vi "UnregisterMat_1DArray-CXT.vi"(6 "AdressOrData":cxt[](array[numeric]), 8 "error in":errorcluster, 11 "Image":u8) -> (0 "error out":errorcluster, 3 "Datatype":cxt[](array[numeric]))   [LabVIEW 2020, in "OpenLvVision_OpenCv.lvlib"]
doc: "Register mat for dll.\nNo malleable to breake vi inlining!"
uses:
  OpenLvVision_OpenCv.lvlib
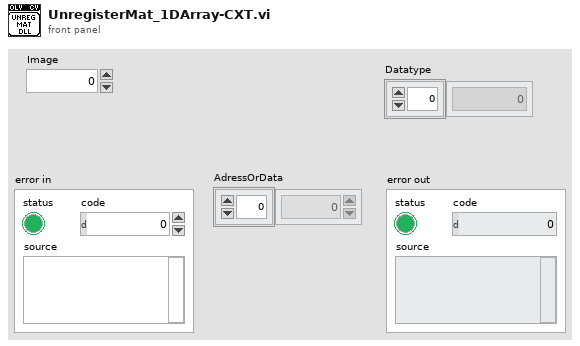
[diagram p1: front panel]
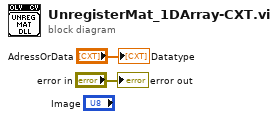
[diagram p0: block diagram]
diagram:
  "error out" <- "error in"
  "Datatype" <- "AdressOrData"
